vi "wireless mode t str.vi"(11 "mode":u32(ring) items=["WIRELESS_PROTO_SYNC", "WIRELESS_PROTO_STREAM", "WIRELESS_PROTO_SPEW", "WIRELESS_PROTO_CARRIER", "WIRELESS_PROTO_CARRIER_SWEEP", "WIRELESS_PROTO_STREAM_MUX", "WIRELESS_PROTO_SUPER_SPEW", "WIRELESS_PROTO_CONFIG", "WIRELESS_PROTO_CLOCK_CAL", "WIRELESS_PROTO_ACCESS_POINT"]) -> (3 "function return":string)   [LabVIEW 2019, in "apdm.lvlib"]
doc: "APDM_EXPORT const char* apdm_wireless_mode_t_str(const apdm_wireless_mode_t mode);"
uses:
  apdm.lvlib
  Lee Lab/CP FES Walking 2018/Code/Working/LabVIEW/apdm.dll
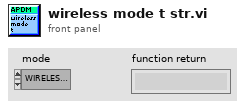
[diagram p1: front panel]
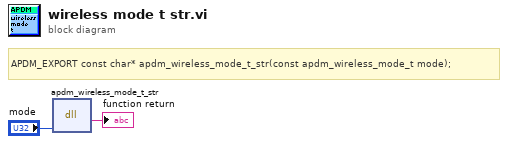
[diagram p0: block diagram]
diagram:
  # "APDM_EXPORT const char* apdm_wireless_mode_t_str(const apdm_wireless_mode_t mode);"
  n1 = dll-call lib="C:/Users/jfalesi/Dropbox/Lee Lab/CP FES Walking 2018/Code/Working/LabVIEW/apdm.*" fn="apdm_wireless_mode_t_str"("mode"="mode") -> (→"function return":string)  [unwired: 4 in, 2 out]
